vi "GUI Select or Deselect all BPM or PS.vi"(8 "error in (no error)":errorcluster, 10 "Boolean Value":bool, 11 "Variable Selector In":T1[](array[typedef])) -> (0 "error out":errorcluster, 3 "Variable Selector Out":T1[](array[typedef]))   [LabVIEW 2011, in "User Interface VIs.lvlib"]
uses:
  User Interface VIs.lvlib
  Types Definitions/Type BPM or PS Selector.ctl
  Type Definitions.lvlib
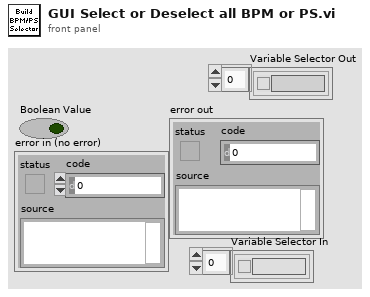
[diagram p1: front panel]
types:
  T1 = typedef "Type Definitions.lvlib/Type BPM or PS Selector.ctl" = cluster{"Name":string, "Active":bool}
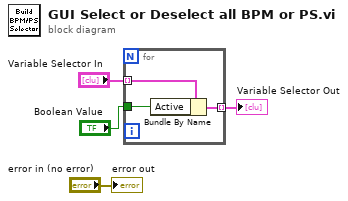
[diagram p0: block diagram]
diagram:
  n1 = for {
    tunnel: "Variable Selector In" -> [w6] mode=indexing
    tunnel: [w7] -> w2 mode=indexing
    tunnel: "Boolean Value" -> [w5]
    n2 = Bundle By Name(cluster=w6, "Active"=w5) -> (w7:T1)
  }
  "Variable Selector Out" <- w2
  "error out" <- "error in (no error)"
